vi "PythonName.vi"(6 "add self":bool, 8 "error in":errorcluster, 11 "FlatSequenceFrame in":refnum<class "FlatSequenceFrame.lvclass">) -> (0 "error out":errorcluster, 3 "FlatSequenceFrame out":refnum<class "FlatSequenceFrame.lvclass">, 5 "name":string, 7 "UID":string)   [LabVIEW 2014, in "FlatSequenceFrame.lvclass"]
uses:
  FlatSequenceFrame.lvclass
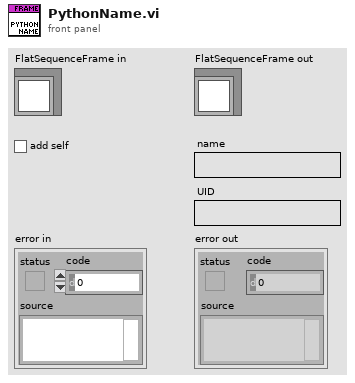
[diagram p1: front panel]
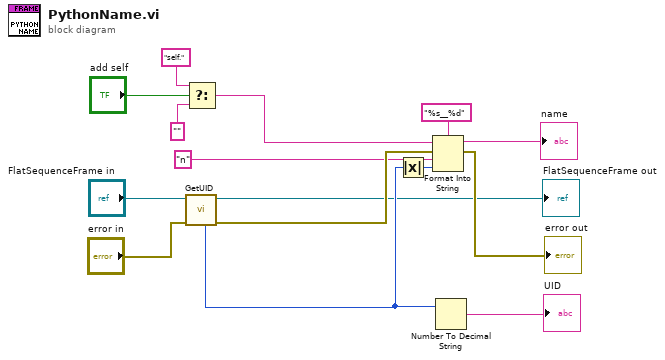
[diagram p0: block diagram]
diagram:
  n1 = call-dynamic "GetUID.vi"("error in"="error in", "FlatSequenceFrame in"="FlatSequenceFrame in") -> ("error out"=w9:errorcluster, "FlatSequenceFrame out"=→"FlatSequenceFrame out":refnum<class "FlatSequenceFrame.lvclass">, "UID"=w10:i32)  [unwired: 5 in]
  n2 = Select(t="self." ("format string"), s="add self", f="") -> (s? t:f=w11:string)
  n3 = Absolute Value(x=w10) -> (abs(x)=w1:i32)
  n4 = Format Into String(format string="%s__%d", initial string=w11, error in=w9, "n" ("input 1"), w1) -> (resulting string=→"name":string, error out=→"error out":errorcluster)
  n5 = Number To Decimal String(number=w10) -> (decimal integer string=→"UID":string)  [unwired: 1 in]
